vi "All Variant to bools.vi"(3 "Error in":errorcluster caption="错误输入", 5 "Variant input":variant[](array[variant])) -> (0 "Error out":errorcluster caption="错误输出", 1 "Var Out":bool[](array[boolean]))   [LabVIEW 2014]
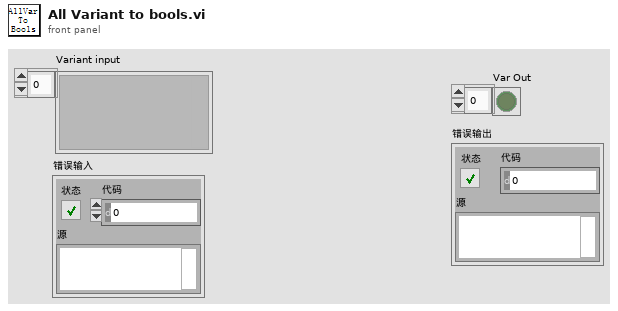
[diagram p1: front panel]
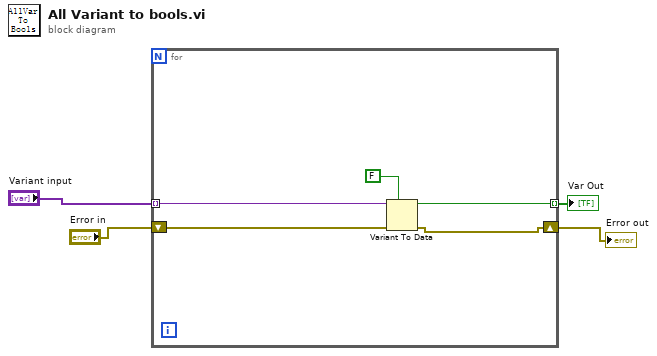
[diagram p0: block diagram]
diagram:
  n1 = for {
    tunnel: "Variant input" -> [w9] mode=indexing
    shift-right: [w7] -> w2
    shift-left: "Error in" -> [w8]
    tunnel: [w5] -> w1 mode=indexing
    n2 = Variant To Data(error in=w8, type=FALSE, Variant=w9) -> (data=w5:bool, error out=w7:errorcluster)
  }
  "Error out" <- w2
  "Var Out" <- w1
